vi "Initialize UI.vi"(8 "error in (no error)":errorcluster, 11 "UI in":refnum<class "UI.lvclass">) -> (0 "error out":errorcluster, 2 "stop event":refnum<user-event>, 3 "UI out":refnum<class "UI.lvclass">)   [LabVIEW 2016, in "Generic UI Actor.lvlib" / "UI.lvclass"]
uses:
  <userlib>/Common Components/User Interface/UI.lvclass
  <userlib>/Common Components/User Interface/UI.lvclass/UI.ctl
  <userlib>/Common Components/User Interface/Accessors/Write This VI.vi
  <userlib>/Common Components/User Interface/Accessors/Read This VI.vi
  <userlib>/Common Components/User Interface/Accessors/Read Hide me.vi
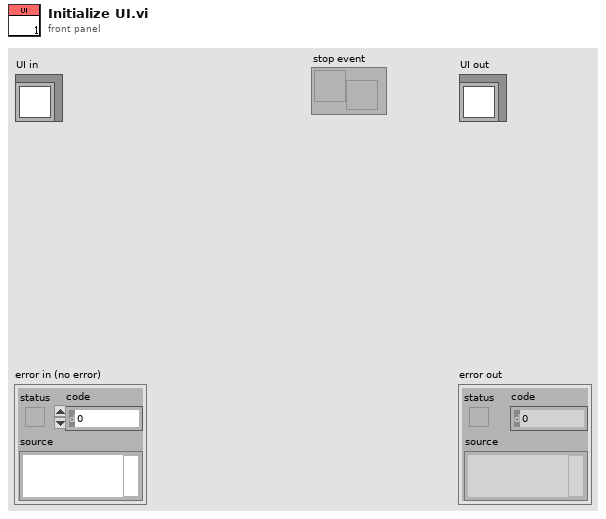
[diagram p1: front panel]
types:
  T1 = enum32{"Invalid", "Standard", "Closed", "Hidden", "Minimized", "Maximized"}
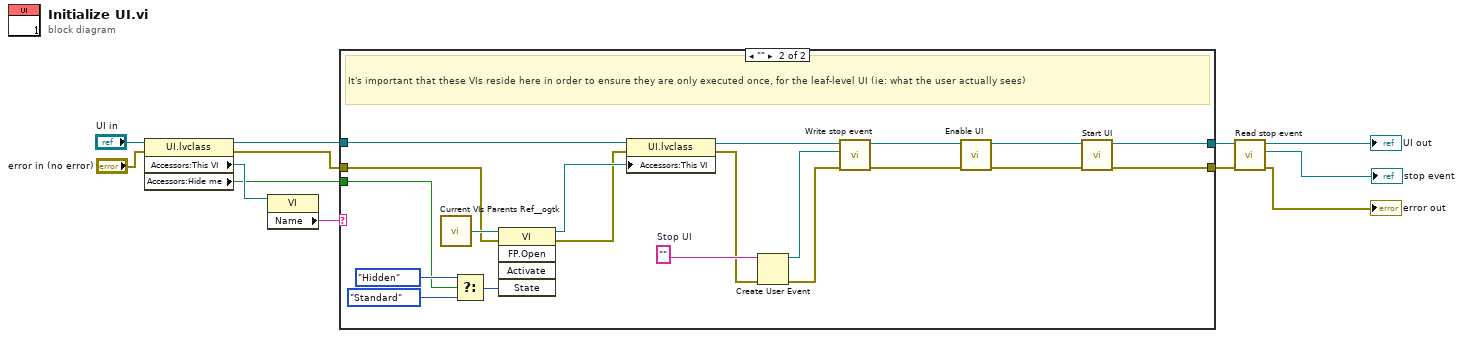
[diagram p0: block diagram]
diagram:
  n1 = property class="UI.lvclass"(reference="UI in", error in="error in (no error)") -> (reference out=w4:refnum<class "UI.lvclass">, error out=w2:errorcluster, "Accessors:This VI"=w3:refnum<vi>, "Accessors:Hide me"=w1:bool)
  n2 = property class="VI"(reference=w3) -> ("Name"=w12:string)  [unwired: 1 in, 2 out]
  n3 = case shown="\"\"" w12 {
    tunnel: [w13 w20] -> w11
    tunnel: w4 -> [w13 w18]
    tunnel: [w14 w21] -> w8
    tunnel: w2 -> [w14 w30]
    tunnel: w1 -> [_ w15]
    frame Default {
    }
    frame "" {
      w31 = ""  # Stop UI
      # "It's important that these VIs reside here in order to ensure they are only executed once, for the leaf-level UI (ie: what the user actually sees)"
      n4 = call <userlib>:"Current VIs Parents Ref__ogtk.vi"() -> ("Calling VI's Reference"=w34:refnum<vi>)  [unwired: 2 in]
      n5 = Select(t=T1."Hidden" ("State"), s=w15, f=T1."Standard" ("State")) -> (s? t:f=w17:T1)
      n6 = invoke class="VI" method="FP.Open"(reference=w34, error in=w30, "State"=w17) -> (reference out=w28:refnum<vi>, error out=w26:errorcluster)  [unwired: 2 in, 3 out]
      n7 = property class="UI.lvclass"(reference=w18, error in=w26, "Accessors:This VI"=w28) -> (reference out=w29:refnum<class "UI.lvclass">, error out=w27:errorcluster)
      n8 = Create User Event(user event datatype=w31, error in=w27) -> (user event=w32:refnum<user-event>, error out=w33:errorcluster)
      n9 = call <userlib>:"Write stop event.vi"("error in (no error)"=w33, "stop event"=w32, "UI in"=w29) -> ("error out"=w24:errorcluster, "UI out"=w25:refnum<class "UI.lvclass">)  [unwired: 7 in]
      n10 = call-dynamic "Enable UI.vi"("error in (no error)"=w24, "UI in"=w25) -> ("error out"=w22:errorcluster, "UI out"=w23:refnum<class "UI.lvclass">)  [unwired: 8 in]
      n11 = call-dynamic "Start UI.vi"("error in (no error)"=w22, "UI in"=w23) -> ("error out"=w21:errorcluster, "UI out"=w20:refnum<class "UI.lvclass">)  [unwired: 8 in]
    }
  }
  n12 = call <userlib>:"Read stop event.vi"("error in (no error)"=w8, "UI in"=w11) -> ("error out"=→"error out":errorcluster, "stop event"=→"stop event":refnum<user-event>, "UI out"=→"UI out":refnum<class "UI.lvclass">)  [unwired: 7 in]
